vi "Create Future Promise Pair.vi"(8 "error in (no error)":errorcluster) -> (0 "error out":errorcluster, 2 "Promise out":refnum<class "Promise.lvclass">, 3 "Future out":refnum<class "Future.lvclass">)   [LabVIEW 2017, in "Futures.lvlib"]
uses:
  Futures.lvlib
  Future/Future.lvclass
  Promise/Promise.lvclass
  Result/Result.lvclass
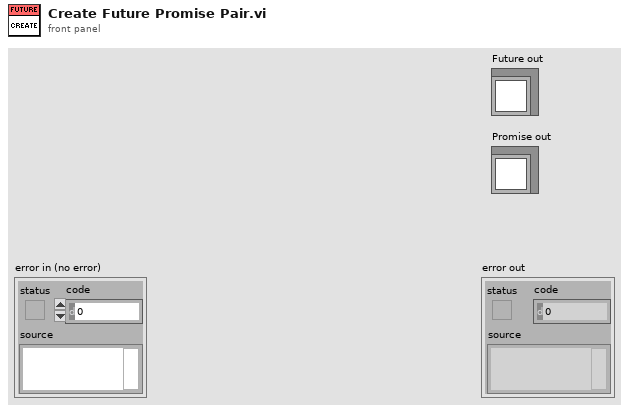
[diagram p1: front panel]
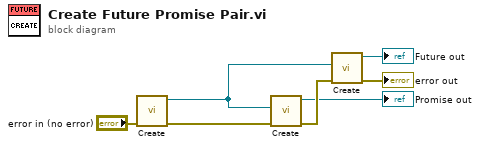
[diagram p0: block diagram]
diagram:
  n1 = call "Create.vi"("error in (no error)"="error in (no error)") -> ("error out"=w5:errorcluster, "Result out"=w7:refnum<class "Result.lvclass">)  [unwired: 9 in]
  n2 = call "Create.vi"("error in (no error)"=w5, "Result"=w7) -> ("error out"=w6:errorcluster, "Promise out"=→"Promise out":refnum<class "Promise.lvclass">)  [unwired: 8 in]
  n3 = call "Create.vi"("error in (no error)"=w6, "Result"=w7) -> ("error out"=→"error out":errorcluster, "Future out"=→"Future out":refnum<class "Future.lvclass">)  [unwired: 8 in]
